vi "Channel String to Number of Channels.vi"(3 "Channels String":string="PXI1Slot2/ai1:3") -> (1 "# channels":i32)   [LabVIEW 2019, in "Instrument.Lockin.lvclass"]
uses:
  Instrument.Lockin.lvclass
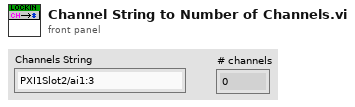
[diagram p1: front panel]
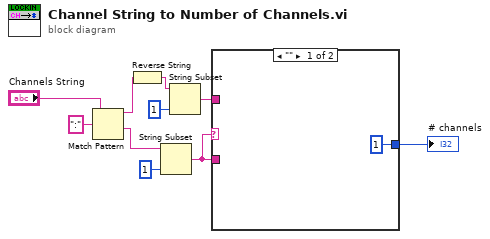
[diagram p0: block diagram]
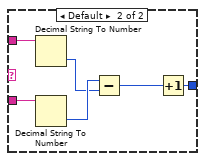
[diagram p2: hidden frame]
diagram:
  n1 = Match Pattern(string="Channels String", regular expression=":") -> (before substring=w4:string, after substring=w5:string)  [unwired: 1 in, 2 out]
  n2 = Reverse String(1:w4) -> (0:w3:string)
  n3 = String Subset(string=w5, length (rest)=1 ("length (rest)")) -> (substring=w1:string)  [unwired: 1 in]
  n4 = String Subset(string=w3, length (rest)=1 ("length (rest)")) -> (substring=w6:string)  [unwired: 1 in]
  n5 = case shown="\"\"" w1 {
    tunnel: w6 -> [_ w17]
    tunnel: w1 -> [_ w16]
    tunnel: [1 w12] -> w2
    frame "" {
    }
    frame Default {
      n6 = Decimal String To Number(string=w17) -> (number=w14:i32)  [unwired: 2 in, 1 out]
      n7 = Decimal String To Number(string=w16) -> (number=w15:i32)  [unwired: 2 in, 1 out]
      n8 = Subtract(x=w15, y=w14) -> (x-y=w13:i32)
      n9 = Increment(x=w13) -> (x+1=w12:i32)
    }
  }
  "# channels" <- w2
